vi "Recall Channel Coefficient.vi"(8 "error in (no error)":errorcluster, 10 "Memory Register (0: A)":i32(ring) items=["A", "B", "C", "D"], 11 "VISA resource name":refnum<visa-resource-name>) -> (0 "error out":errorcluster, 3 "VISA resource name out":refnum<visa-resource-name>)   [LabVIEW 2012, in "Tektronix TTR500 Series.lvlib"]
doc: "Recalls the calibration coefficient for an individual channel from the specified register as the setting of the active channel.\n\nNotes:\n(1) It is possible to recall the register from a different channel where it was saved."
uses:
  <instrlib>/Tektronix TTR500 Series/Tektronix TTR500 Series.lvlib
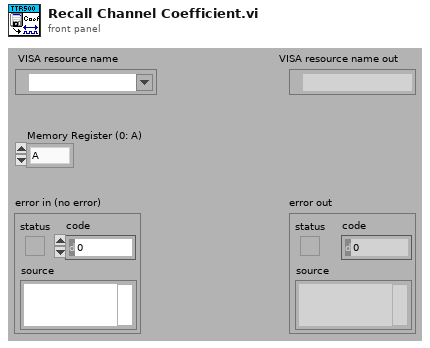
[diagram p1: front panel]
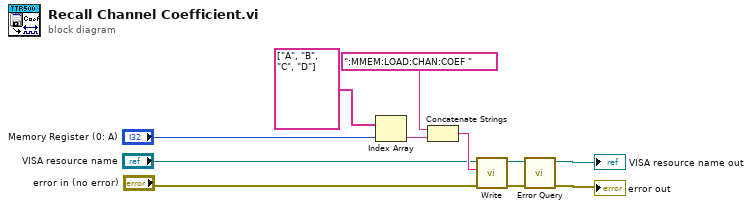
[diagram p0: block diagram]
diagram:
  n1 = Index Array(array=string[] ["A", "B", "C", "D"], index="Memory Register (0: A)") -> (element=w7:string)
  n2 = Concatenate Strings(":MMEM:LOAD:CHAN:COEF ", w7) -> (w5:string)
  n3 = call <instrlib>:"Write.vi"("error in (no error)"="error in (no error)", "String ()"=w5, "VISA resource name"="VISA resource name") -> ("error out"=w3:errorcluster, "VISA resource name out"=w4:refnum<visa-resource-name>)  [unwired: 6 in, 1 out]
  n4 = call <instrlib>:"Error Query.vi"("error in (no error)"=w3, "VISA resource name"=w4) -> ("error out"=→"error out":errorcluster, "VISA resource name out"=→"VISA resource name out":refnum<visa-resource-name>)  [unwired: 6 in, 2 out]
